vi "LSX Get Analog Input.vi"(8 "error in (no error)":errorcluster, 9 "plValue":i32, 10 "lIndex":i32, 11 "lLSID":i32) -> (0 "error out":errorcluster, 1 "plValue out":i32, 3 "function return":i32)   [LabVIEW 2018, in "Tango.lvlib"]
doc: "TANGOAPI int TANGOCALL LSX_GetAnalogInput (int lLSID, int lIndex, int *plValue);"
uses:
  <userlib>/Tango/Tango.lvlib
  <userlib>/Tango/Tango_DLL.dll
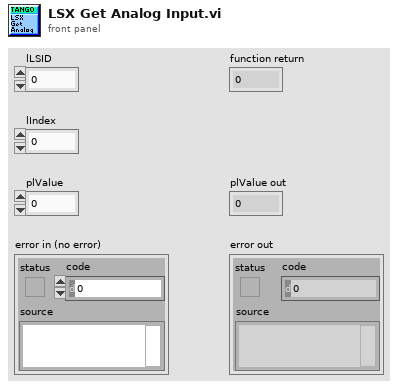
[diagram p1: front panel]
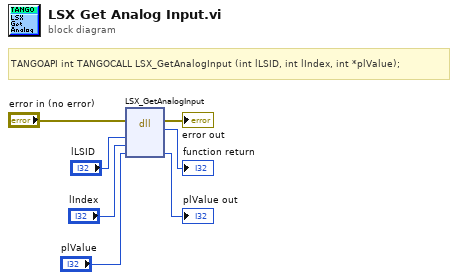
[diagram p0: block diagram]
diagram:
  # "TANGOAPI int TANGOCALL LSX_GetAnalogInput (int lLSID, int lIndex, int *plValue);"
  n1 = dll-call lib="C:/Program Files (x86)/National Instruments/LabVIEW 2018/user.lib/Tango/Tango_DLL.*" fn="LSX_GetAnalogInput"(error in="error in (no error)", "lLSID"="lLSID", "lIndex"="lIndex", "plValue"="plValue") -> (error out=→"error out":errorcluster, →"function return":i32, "plValue"=→"plValue out":i32)  [unwired: 4 in, 1 out]
